vi "HovaCAL start flow.vi"(8 "error in (no error)":errorcluster caption="Fehler (Eingang, kein Fehler)", 10 "run":bool, 11 "total flow setpoint":dbl) -> (0 "error out":errorcluster caption="Fehler (Ausgang)")   [LabVIEW 2020, in "EPA 1065.lvlib" / "HovaCAL Interference verificaton.lvlib"]
uses:
  HovaCAL Interference verificaton.lvlib
  Linearisierung V2/Gasteiler/HovaCAL_Interface/Kommunikation/Kommunikation.lvlib
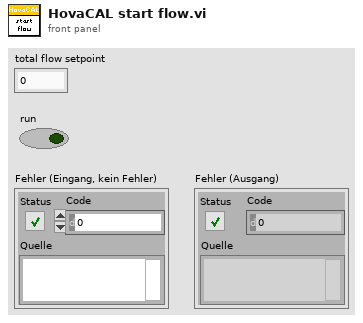
[diagram p1: front panel]
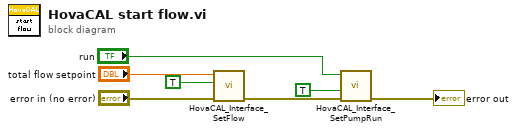
[diagram p0: block diagram]
diagram:
  n1 = call "HovaCAL_Interface_SetFlow.vi"("error in (no error)"="error in (no error)", "sofort"=TRUE, "total flow setpoint"="total flow setpoint") -> ("error out"=w3:errorcluster)  [unwired: 8 in]
  n2 = call "HovaCAL_Interface_SetPumpRun.vi"("error in (no error)"=w3, "sofort"=TRUE, "run"="run") -> ("error out"=→"error out":errorcluster)  [unwired: 8 in]
